vi "PLC.WriteDataBlock.vi"(8 "error in (no error)":errorcluster, 9 "data in":u8[](array[numeric]) format="%02x", 10 "Block":i32, 11 "Ref":u64) -> (0 "error out":errorcluster, 3 "ref out":u64)   [LabVIEW 2016]
doc: "WriteDataBlock\n\nWabco 2017 All right reserved\nAuthor: maciej.szupienko@wabco-auto.com"
uses:
  Snap7/lib/Snap7.lvlib
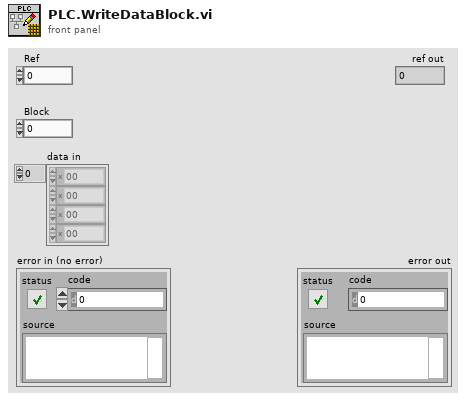
[diagram p1: front panel]
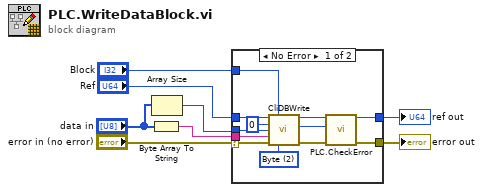
[diagram p0: block diagram]
diagram:
  n1 = Byte Array To String(unsigned byte array="data in") -> (string=w3:string)
  n2 = Array Size(array="data in") -> (size(s)=w4:i32)
  n3 = case shown="No Error" "error in (no error)" {
    selector: "error in (no error)" -> [w15 w21]
    tunnel: [w12 w21] -> w8
    tunnel: [w19 w20] -> w7
    tunnel: w4 -> [w17 _]
    tunnel: "Ref" -> [w16 w20]
    tunnel: w3 -> [w14 _]
    tunnel: "Block" -> [w10 _]
    frame No Error {
      w18 = 2 items=["Bit"=1, "Byte"=2, "Word"=4, "DWord"=6, "Real"=8, "Counter"=28, "Timer"=29] ("Word Length")
      n4 = call "CliDBWrite.vi"("ref in"=w16, "DB Number"=w10, "Start"=0, "Amount"=w17, "data in"=w14, "error in (no error)"=w15, "Word Length"=w18) -> ("ref out"=w19:u64, "Result"=w11:i32, "error out"=w13:errorcluster)  [unwired: 6 in]
      n5 = call "PLC.CheckError.vi"("error in (no error)"=w13, "Result"=w11) -> ("error out"=w12:errorcluster)  [unwired: 9 in]
    }
    frame Error {
    }
  }
  "error out" <- w8
  "ref out" <- w7
